vi "EXDIR-YAML_Recursive_YAML_Lines_to_Dictionary.vi"(9 "End Index":i32, 10 "Start Index":i32, 11 "ENTIRE Array of YAML Lines":string[](array[string])) -> (1 "dictionary out":T1, 2 "created new?":bool, 3 "Dictionary Items":cluster{"key":variant, "value":variant}[](array[cluster]))   [LabVIEW 2016]
uses:
  <userlib>/_OpenG.lib/dictionary/dictionary.llb/Dictionary Object RefNum__ogtk.ctl
  <userlib>/_OpenG.lib/dictionary/dictionary.llb/Dictionary Object RefNum - Enum__ogtk.ctl
  <userlib>/_OpenG.lib/dictionary/dictionary.llb/Dictionary Update (by scalar value)__ogtk.vi
panel:
  out "Numeric":i32
  out "while loop iter":i32
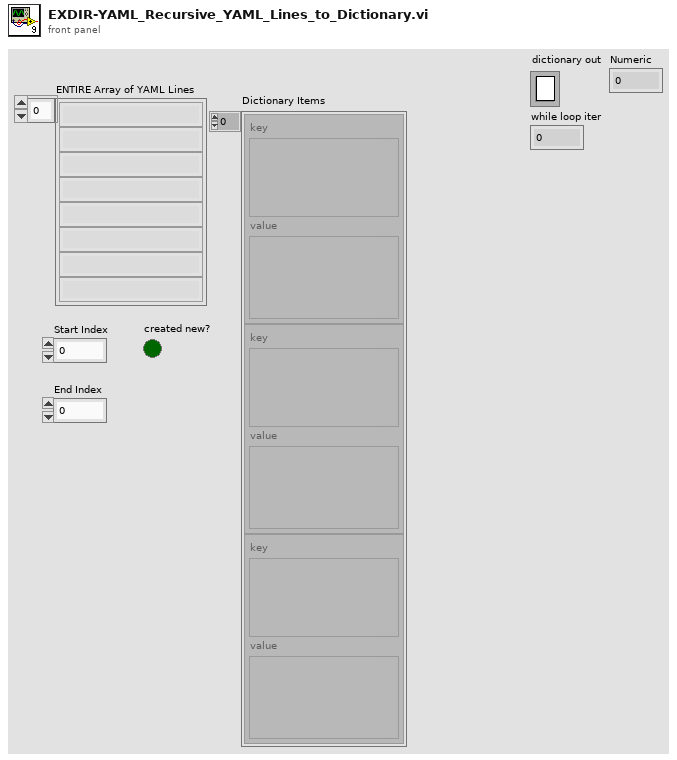
[diagram p1: front panel]
types:
  T1 = typedef "Dictionary Object RefNum__ogtk.ctl" = refnum<k1>
  T2 = cluster{string, "Dictionary Items":cluster{"key":variant, "value":variant}[]}
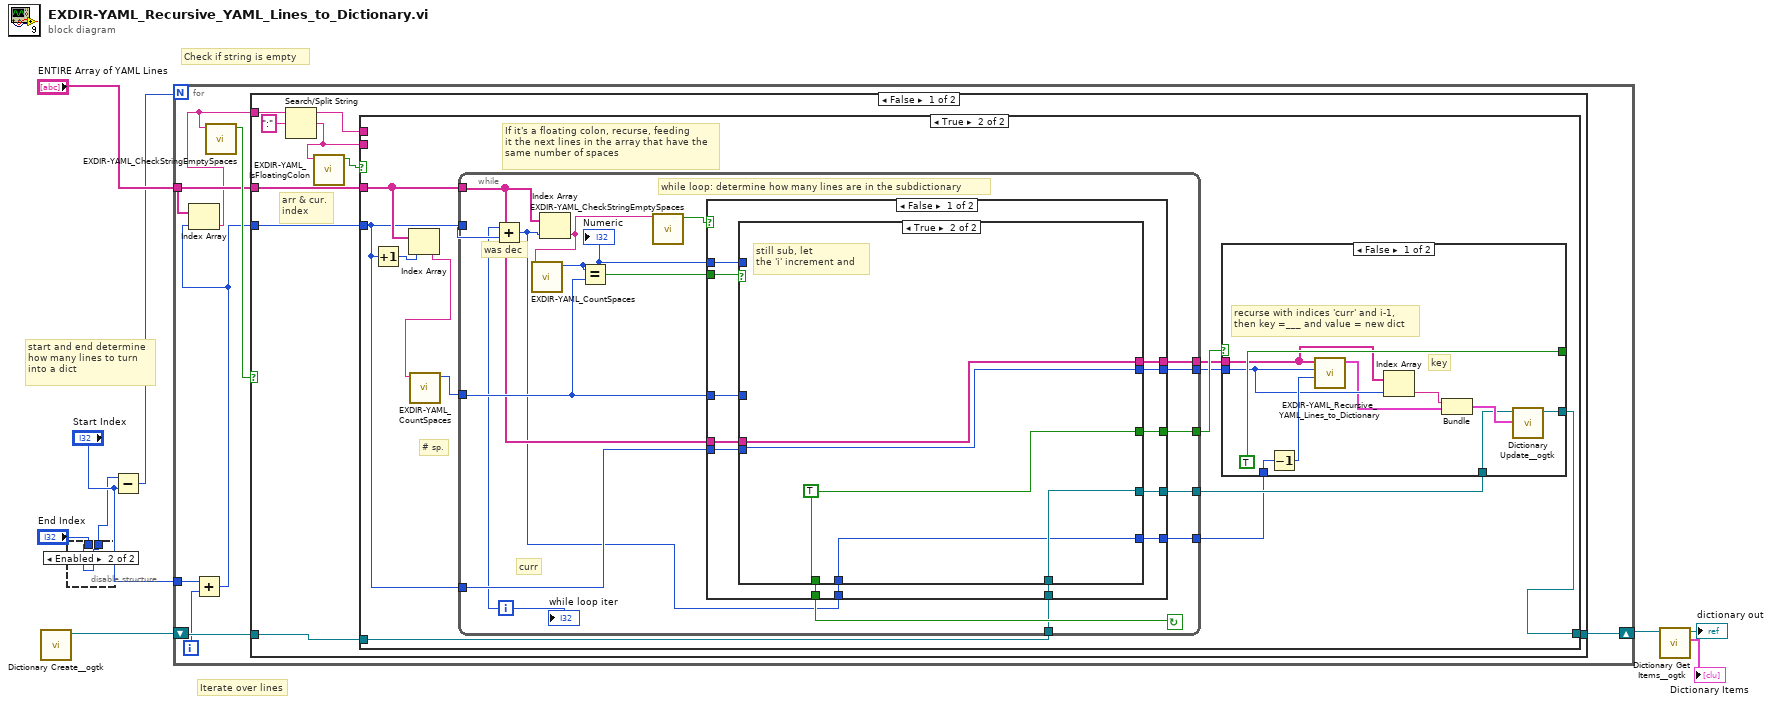
[diagram p0: block diagram]
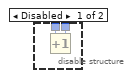
[diagram p2: hidden frame]
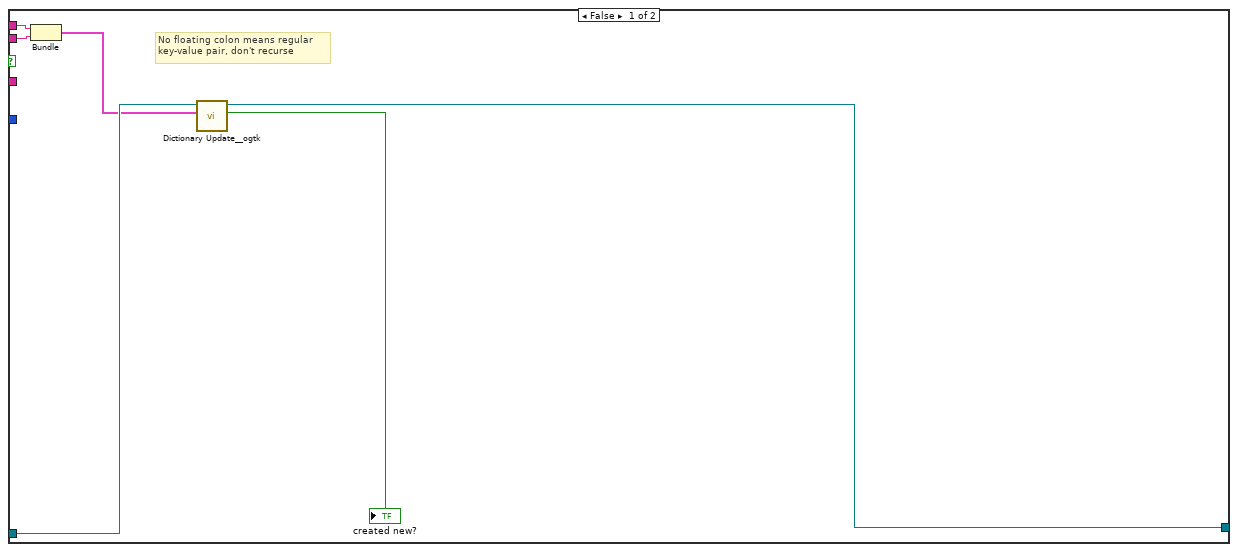
[diagram p3: hidden frame]
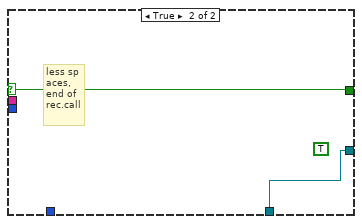
[diagram p4: hidden frame]
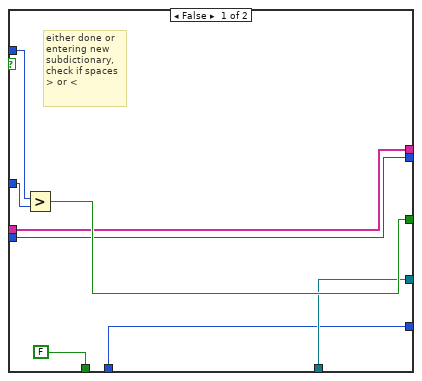
[diagram p5: hidden frame]
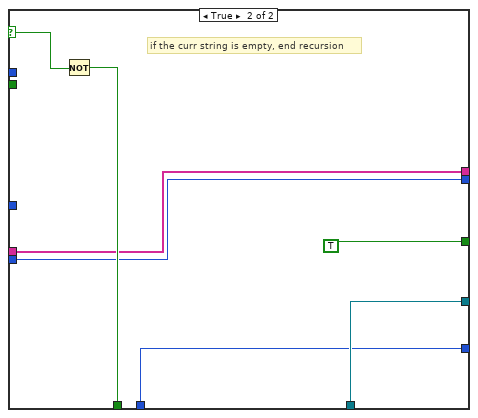
[diagram p6: hidden frame]
diagram:
  # "start and end determine\nhow many lines to turn\ninto a dict"
  # "Iterate over lines"
  # "Check if string is empty"
  n1 = call <userlib>:"Dictionary Create__ogtk.vi"() -> ("dictionary out"=w7:T1)  [unwired: 10 in, 1 out]
  n2 = disable-structure shown="Enabled" {
    disable-tunnel: "End Index" -> [w11 w12]
    disable-tunnel: [w10 w12] -> w1
    frame Disabled {
      n3 = Increment(x=w11) -> (x+1=w10:i32)
    }
    frame Enabled {
    }
  }
  n4 = Subtract(x=w1, y="Start Index") -> (x-y=w4:i32)
  n5 = for {
    N: w4 -> [_]
    shift-right: [w19] -> w8
    shift-left: w7 -> [w20]
    tunnel: "ENTIRE Array of YAML Lines" -> [w15]
    tunnel: "Start Index" -> [w16]
    i -> [w17]
    n6 = Add(x=w16, y=w17) -> (x+y=w14:i32)
    n7 = Index Array(array=w15, index=w14) -> (element=w13:string)
    n8 = call "EXDIR-YAML_CheckStringEmptySpaces.vi"("String"=w13) -> ("empty or all spaces"=w18:bool)  [unwired: 10 in]
    n9 = case shown="False" w18 {
      tunnel: w13 -> [w29 _]
      tunnel: w20 -> [w27 w110]
      tunnel: [w25 w110] -> w19
      tunnel: w15 -> [w22 _]
      tunnel: w14 -> [w21 _]
      frame False {
        # "arr & cur.\nindex"
        n10 = Search/Split String(string=w29, search string/char (-)=":") -> (substring before match=w26:string, match + rest of string=w24:string)  [unwired: 1 in, 1 out]
        n11 = call "EXDIR-YAML_IsFloatingColon.vi"("String"=w24) -> ("after the 1st char is empty or all spaces"=w23:bool)  [unwired: 10 in]
        n12 = case shown="True" w23 {
          tunnel: w27 -> [w35 w42]
          tunnel: w26 -> [w34 _]
          tunnel: [w31 w37] -> w25
          tunnel: w24 -> [w30 _]
          tunnel: w22 -> [_ w46]
          tunnel: w21 -> [_ w43]
          frame False {
            # "No floating colon means regular\nkey-value pair, don't recurse"
            n13 = Bundle(w34, w30) -> (w33:cluster{string, string})  [unwired: 1 in]
            n14 = call-poly <userlib>:"Dictionary Update__ogtk.vi"("key-value"=w33, "dictionary"=w35) -> ("created new?"=→"created new?":bool, "dictionary out"=w31:T1)  [unwired: 7 in, 1 out]
          }
          frame True {
            # "# sp."
            # "If it's a floating colon, recurse, feeding\nit the next lines in the array that have the\nsame number of spaces"
            n15 = Increment(x=w43) -> (x+1=w47:i32)
            n16 = Index Array(array=w46, index=w47) -> (element=w45:string)
            n17 = call "EXDIR-YAML_CountSpaces.vi"("String"=w45) -> ("Numeric"=w44:i32)  [unwired: 10 in]
            n18 = while {
              tunnel: w46 -> [w70]
              tunnel: w43 -> [w76]
              tunnel: w44 -> [w73]
              tunnel: w43 -> [w71]
              tunnel: w42 -> [w69]
              tunnel: [w68] -> w38
              tunnel: [w63] -> w41
              tunnel: [w62] -> w40
              tunnel: [w61] -> w39
              tunnel: [w60] -> w36
              i -> [w65]
              stop <- w72 continue-if-true
              # "while loop: determine how many lines are in the subdictionary"
              # "was dec"
              # "curr"
              n19 = Add(x=w65, y=w76) -> (x+y=w64:i32)
              n20 = Index Array(array=w70, index=w64) -> (element=w67:string)
              n21 = call "EXDIR-YAML_CountSpaces.vi"("String"=w67) -> ("Numeric"=w74:i32)  [unwired: 10 in]
              "Numeric" <- w74
              n22 = Equal?(x=w74, y=w73) -> (x = y?=w75:bool)
              n23 = call "EXDIR-YAML_CheckStringEmptySpaces.vi"("String"=w67) -> ("empty or all spaces"=w66:bool)  [unwired: 10 in]
              n24 = case shown="False" w66 {
                selector: w66 -> [_ w109]
                tunnel: w75 -> [w89 _]
                tunnel: w74 -> [w88 _]
                tunnel: w73 -> [w87 _]
                tunnel: [w86 w107] -> w72
                tunnel: w71 -> [w85 w104]
                tunnel: w70 -> [w84 w105]
                tunnel: w69 -> [w83 w108]
                tunnel: [w82 w108] -> w68
                tunnel: w64 -> [w81 w103]
                tunnel: [w80 TRUE] -> w63
                tunnel: [w79 w105] -> w62
                tunnel: [w78 w104] -> w61
                tunnel: [w77 w103] -> w60
                frame False {
                  n25 = case shown="True" w89 {
                    tunnel: w88 -> [w97 _]
                    tunnel: w87 -> [w96 _]
                    tunnel: [FALSE w99] -> w86
                    tunnel: w81 -> [w90 w98]
                    tunnel: w85 -> [w92 w100]
                    tunnel: w84 -> [w93 w101]
                    tunnel: w83 -> [w91 w102]
                    tunnel: [w91 w102] -> w82
                    tunnel: [w94 w99] -> w80
                    tunnel: [w93 w101] -> w79
                    tunnel: [w92 w100] -> w78
                    tunnel: [w90 w98] -> w77
                    frame False {
                      # "either done or\nentering new\nsubdictionary,\ncheck if spaces\n> or <"
                      n26 = Greater?(x=w97, y=w96) -> (0:w94:bool)
                    }
                    frame True {
                      w99 = TRUE
                      # "still sub, let \nthe 'i' increment and"
                    }
                  }
                }
                frame True {
                  # "if the curr string is empty, end recursion"
                  n27 = Not(x=w109) -> (.not. x?=w107:bool)
                }
              }
              "while loop iter" <- w65
            }
            n28 = case shown="False" w41 {
              selector: w41 -> [_ w59]
              tunnel: [TRUE w59] -> _
              tunnel: w36 -> [w56 _]
              tunnel: w39 -> [w54 _]
              tunnel: w40 -> [w53 _]
              tunnel: w38 -> [w50 w58]
              tunnel: [w49 w58] -> w37
              frame False {
                # "key"
                # "recurse with indices 'curr' and i-1,\nthen key =___ and value = new dict"
                n29 = Decrement(x=w56) -> (x-1=w55:i32)
                n30 = call "EXDIR-YAML_Recursive_YAML_Lines_to_Dictionary.vi"("End Index"=w55, "Start Index"=w54, "ENTIRE Array of YAML Lines"=w53) -> ("Dictionary Items"=w48:cluster{"key":variant, "value":variant}[])  [unwired: 6 in, 2 out]
                n31 = Index Array(array=w53, index=w54) -> (element=w52:string)
                n32 = Bundle(w52, "Dictionary Items"=w48) -> (w51:T2)  [unwired: 1 in]
                n33 = call-poly <userlib>:"Dictionary Update__ogtk.vi"("key-value"=w51, "dictionary"=w50) -> ("dictionary out"=w49:T1)  [unwired: 7 in, 2 out]
              }
              frame True {
                (unwired) TRUE
                # "less sp\naces,\nend of\nrec.call"
              }
            }
          }
        }
      }
      frame True {
        # "if it's an empty line, ignore it"
      }
    }
  }
  n34 = call <userlib>:"Dictionary Get Items__ogtk.vi"("dictionary"=w8) -> ("items"=→"Dictionary Items":cluster{"key":variant, "value":variant}[], "dictionary out"=→"dictionary out":T1)  [unwired: 8 in, 1 out]
